vi "basic_functions.vi"() -> ()   [LabVIEW 2019]
panel:
  out "Array Output":dbl[][](array[numeric])
  in  "Numeric":dbl
  in  "Array Input":dbl[][](array[numeric])
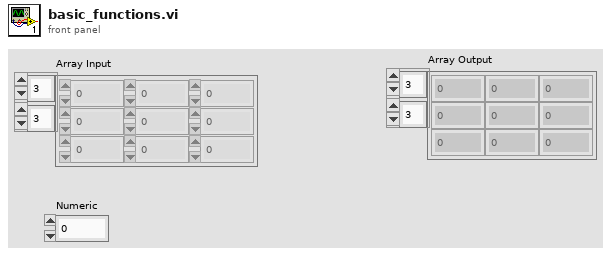
[diagram p1: front panel]
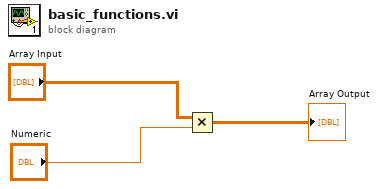
[diagram p0: block diagram]
diagram:
  n1 = Multiply(x="Array Input", y="Numeric") -> (x*y=→"Array Output":dbl[][])
